vi "UpdateDataToMeter.vi"(1 "SelectedDeviceChannelsData":T1[](array[typedef]), 9 "ProcessMeterRef":refnum<vi>[](array[refnum])) -> ()   [LabVIEW 2010]
uses:
  Ctrls/ChannelData.ctl
  Ctrls/ChannelType.ctl
  Ctrls/ChannelAccessType.ctl
  Ctrls/Precess Meter.ctl
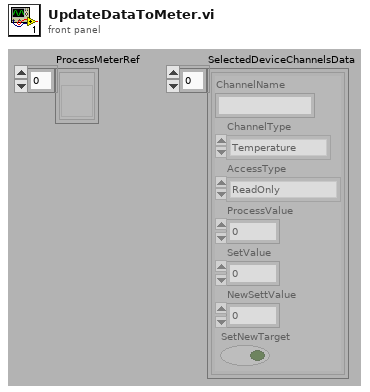
[diagram p1: front panel]
types:
  T1 = typedef "ChannelData.ctl" = cluster{"ChannelName":string, "ChannelType":T2, "AccessType":T3, "ProcessValue":dbl, "SetValue":dbl, "NewSettValue":dbl, "SetNewTarget":bool}
  T2 = typedef "ChannelType.ctl" = enum16{"Temperature", "Humidity"}
  T3 = typedef "ChannelAccessType.ctl" = enum16{"ReadOnly", "SetTarget"}
  T4 = typedef "Precess Meter.ctl" = cluster{"当前值":dbl, "设定值":dbl, "通道选择":string, "设置设定值":bool, "显示曲线":bool}
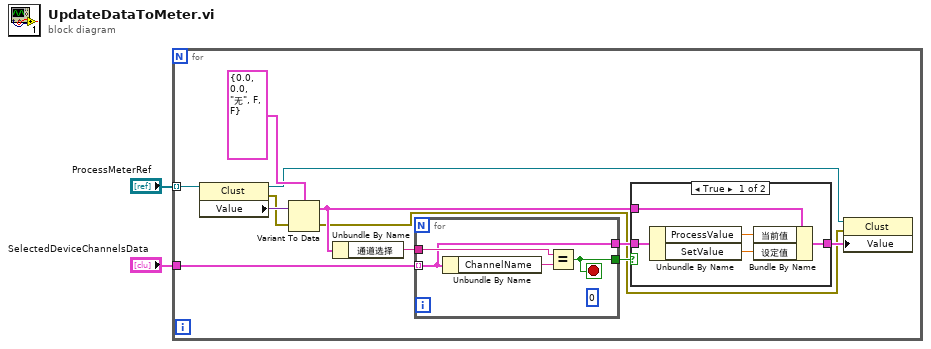
[diagram p0: block diagram]
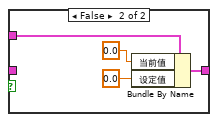
[diagram p2: hidden frame]
diagram:
  n1 = for {
    tunnel: "ProcessMeterRef" -> [w14] mode=indexing
    tunnel: "SelectedDeviceChannelsData" -> [w11]
    n2 = property class="Clust"(reference=w14) -> (reference out=w6:refnum<vi>, error out=w4:errorcluster, "Value"=w13:variant)  [unwired: 1 in]
    n3 = Variant To Data(error in=w4, Variant=w13, type=T4 {"当前值"=0.0, "设定值"=0.0, "通道选择"="无", "设置设定值"=FALSE, "显示曲线"=FALSE} ("ProcessMeter 1")) -> (error out=w3:errorcluster, data=w7:T4)
    n4 = Unbundle By Name(w7) -> ("通道选择"=w10:string)
    n5 = for {
      tunnel: w11 -> [w24] mode=indexing
      tunnel: w10 -> [w26]
      tunnel: [w25] -> w9
      tunnel: [w24] -> w8
      stop <- w25 stop-if-true
      (unwired) 0
      n6 = Unbundle By Name(w24) -> ("ChannelName"=w27:string)
      n7 = Equal?(x=w26, y=w27) -> (x = y?=w25:bool)
    }
    n8 = case shown="True" w9 {
      tunnel: w8 -> [w18 _]
      tunnel: w7 -> [w19 w23]
      tunnel: [w17 w22] -> w5
      frame True {
        n9 = Unbundle By Name(w18) -> ("ProcessValue"=w16:dbl, "SetValue"=w15:dbl)
        n10 = Bundle By Name(cluster=w19, "当前值"=w16, "设定值"=w15) -> (w17:T4)
      }
      frame False {
        n11 = Bundle By Name(cluster=w23, "当前值"=0.0, "设定值"=0.0) -> (w22:T4)
      }
    }
    n12 = property class="Clust"(reference=w6, error in=w3, "Value"=w5) -> ()  [unwired: 2 out]
  }
